vi "Run Till Abort TESTES.vi"() -> ()   [LabVIEW 2012]
uses:
  CCDCamera/CCDCamera.lvclass
  <userlib>/atmcd32d.llb/TriggerMode_mode typedef.ctl
  <userlib>/atmcd32d.llb/HSSpeed_type typedef.ctl
  <userlib>/atmcd32d.llb/Shutter_type typedef.ctl
  <userlib>/atmcd32d.llb/Shutter_mode typedef.ctl
  <userlib>/atmcd32d.llb/ReadMode_mode typedef.ctl
  <userlib>/atmcd32d.llb/AcquisitionMode_mode typedef.ctl
panel:
  out "exposure":sgl format="%.2f"
  out "kinetic":sgl format="%.2f"
  in  "stop":bool
  out "size(s) 2":i32
  out "index":i32
  out "array":u16[](array[numeric])
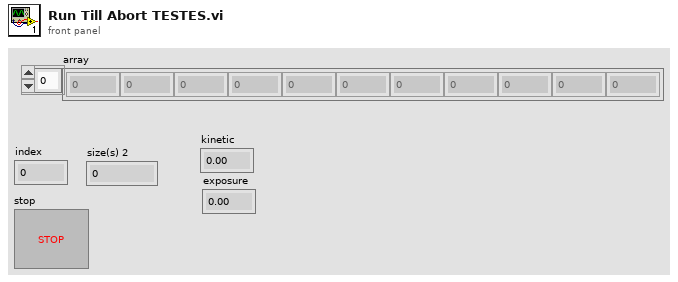
[diagram p1: front panel]
types:
  T1 = typedef "ReadMode_mode typedef.ctl" = enum16{"Full Vertical Binning", "Multi-Track", "Random-Track", "Single-Track", "Image"}
  T2 = typedef "Shutter_mode typedef.ctl" = enum16{"Auto", "Open", "Close", "N/A (3)", "Open FVB Series", "Open Any Series"}
  T3 = typedef "Shutter_type typedef.ctl" = enum16{"TTL Low", "TTL High"}
  T4 = typedef "HSSpeed_type typedef.ctl" = enum16{"EM Amp", "Conventional Amp"}
  T5 = typedef "TriggerMode_mode typedef.ctl" = enum16{"Internal", "External", "N/A (2)", "N/A (3)", "N/A (4)", "N/A (5)", "External Start", "External Exposure (Bulb)", "N/A (8)", "External FVB EM", "Software", "N/A (11)", "External Charge Shifting"}
  T6 = typedef "AcquisitionMode_mode typedef.ctl" = enum16{"Reserved (0)", "Single Scan", "Accumulate", "Kinetics", "Fast Kinetics", "Run Till Abort", "Reserved (6)", "Reserved (7)", "Reserved (8)", "Time Delayed Integration"}
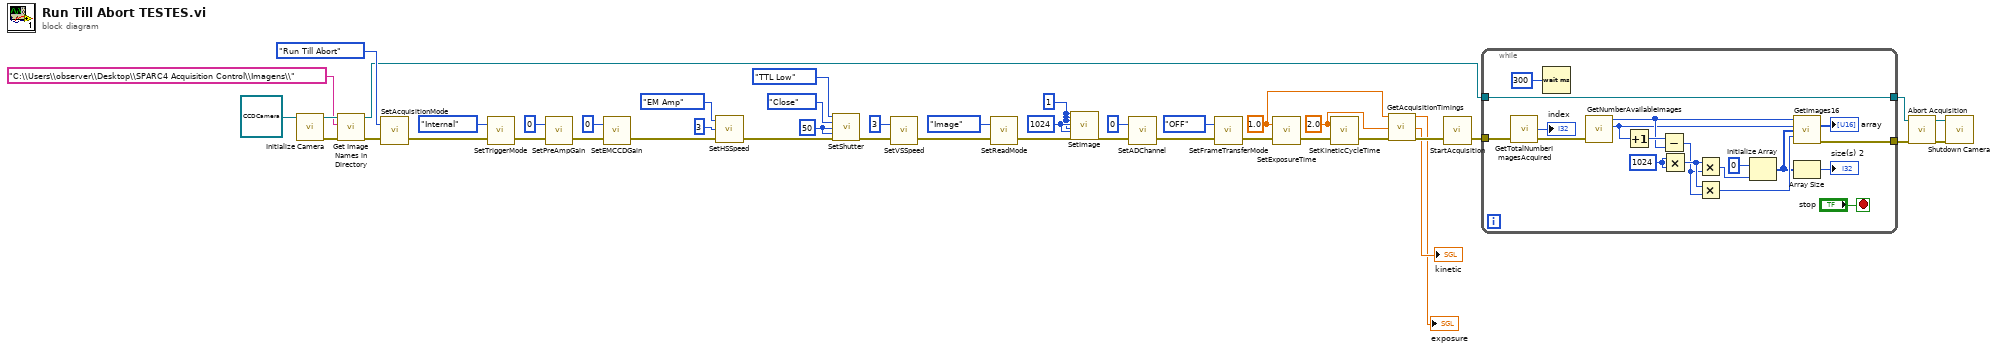
[diagram p0: block diagram]
diagram:
  w3 = sgl 2.0 ("kinetic input")
  w4 = sgl 1.0 ("exposure input")
  w21 = 1024 ("hbin")
  w14 = 1 ("hbin")
  w24 = 50 ("closingtime")
  n1 = call "Initialize Camera.vi"("CCDCamera in"=refnum<class "CCDCamera.lvclass"> refnum) -> ("error out"=w18:errorcluster, "CCDCamera out"=w17:refnum<class "CCDCamera.lvclass">)  [unwired: 9 in]
  n2 = call "Get Image Names in Directory.vi"("error in (no error)"=w18, "Image Path"="C:\\Users\\observer\\Desktop\\SPARC4 Acquisition Control\\Imagens\\", "CCDCamera in"=w17) -> ("error out"=w15:errorcluster, "CCDCamera out"=w12:refnum<class "CCDCamera.lvclass">)  [unwired: 7 in]
  n3 = call <userlib>:"SetAcquisitionMode.vi"("error in (no error)"=w15, "mode"=AcquisitionMode_mode_typedef."Run Till Abort") -> ("error out"=w42:errorcluster)  [unwired: 1 out]
  n4 = call <userlib>:"SetTriggerMode.vi"("error in (no error)"=w42, "mode"=TriggerMode_mode_typedef."Internal") -> ("error out"=w36:errorcluster)  [unwired: 1 out]
  n5 = call <userlib>:"SetPreAmpGain.vi"("error in (no error)"=w36, "index"=0) -> ("error out"=w34:errorcluster)  [unwired: 1 out]
  n6 = call <userlib>:"SetEMCCDGain.vi"("error in (no error)"=w34, "gain"=0) -> ("error out"=w35:errorcluster)  [unwired: 1 out]
  n7 = call <userlib>:"SetHSSpeed.vi"("error in (no error)"=w35, "index"=3, "type"=HSSpeed_type_typedef."EM Amp") -> ("error out"=w37:errorcluster)  [unwired: 1 in, 1 out]
  n8 = call <userlib>:"SetShutter.vi"("type"=Shutter_type_typedef."TTL Low", "mode"=Shutter_mode_typedef."Close", "closingtime"=w24, "openingtime"=w24, "error in (no error)"=w37) -> ("error out"=w41:errorcluster)  [unwired: 9 in, 1 out]
  n9 = call <userlib>:"SetVSSpeed.vi"("error in (no error)"=w41, "index"=3) -> ("error out"=w40:errorcluster)  [unwired: 1 out]
  n10 = call <userlib>:"SetReadMode.vi"("error in (no error)"=w40, "mode"=ReadMode_mode_typedef."Image") -> ("error out"=w39:errorcluster)  [unwired: 1 out]
  n11 = call <userlib>:"SetImage.vi"("hbin"=w14, "vbin"=w14, "hstart"=w14, "hend"=w21, "vstart"=w14, "vend"=w21, "error in (no error)"=w39) -> ("error out"=w38:errorcluster)  [unwired: 19 in, 1 out]
  n12 = call <userlib>:"SetADChannel.vi"("error in (no error)"=w38, "channel"=0) -> ("error out"=w33:errorcluster)  [unwired: 1 out]
  n13 = call <userlib>:"SetFrameTransferMode.vi"("error in (no error)"=w33, "mode"=enum16{"OFF", "ON"}."OFF") -> ("error out"=w13:errorcluster)  [unwired: 1 out]
  n14 = call <userlib>:"SetExposureTime.vi"("error in (no error)"=w13, "time"=w4) -> ("error out"=w19:errorcluster)  [unwired: 1 out]
  n15 = call <userlib>:"SetKineticCycleTime.vi"("error in (no error)"=w19, "time"=w3) -> ("error out"=w6:errorcluster)  [unwired: 1 out]
  n16 = call <userlib>:"GetAcquisitionTimings.vi"("exposure input"=w4, "kinetic input"=w3, "error in (no error)"=w6) -> ("exposure"=→"exposure":sgl, "kinetic"=→"kinetic":sgl, "error out"=w5:errorcluster)  [unwired: 8 in, 2 out]
  n17 = call <userlib>:"StartAcquisition.vi"("error in (no error)"=w5) -> ("error out"=w9:errorcluster)  [unwired: 1 in, 1 out]
  n18 = while {
    tunnel: w9 -> [w62]
    tunnel: [w60] -> w8
    tunnel: w12 -> [w60]
    tunnel: [w54] -> w7
    stop <- "stop" stop-if-true
    w56 = 1024
    n19 = call <userlib>:"GetTotalNumberImagesAcquired.vi"("error in (no error)"=w62) -> ("error out"=w55:errorcluster, "index"=→"index":i32)  [unwired: 2 in, 1 out]
    n20 = Wait (ms)(milliseconds to wait=u32 300) -> ()  [unwired: 1 out]
    n21 = call <userlib>:"GetNumberAvailableImages.vi"("error in (no error)"=w55) -> ("first"=w47:i32, "last"=w46:i32)  [unwired: 2 in, 2 out]
    n22 = Increment(x=w46) -> (x+1=w57:i32)
    n23 = Subtract(x=w57, y=w47) -> (x-y=w45:i32)
    n24 = Multiply(x=w56, y=w56) -> (x*y=w53:i32)
    n25 = Multiply(x=w53, y=w45) -> (x*y=w51:i32)
    n26 = Multiply(x=w53, y=w45) -> (x*y=w58:i32)
    n27 = Initialize Array(u16 0, w51) -> (w50:u16[])
    n28 = call <userlib>:"GetImages16.vi"("first"=w47, "last"=w46, "array"=w50, "size"=w58) -> ("array"=→"array":u16[], "error out"=w54:errorcluster)  [unwired: 7 in, 3 out]
    n29 = Array Size(array=w50) -> (size(s)=→"size(s) 2":i32)
  }
  n30 = call "Abort Acquisition.vi"("error in (no error)"=w7, "CCDCamera in"=w8) -> ("error out"=w10:errorcluster, "CCDCamera out"=w11:refnum<class "CCDCamera.lvclass">)  [unwired: 8 in]
  n31 = call "Shutdown Camera.vi"("error in (no error)"=w10, "CCDCamera in"=w11) -> ()  [unwired: 8 in, 2 out]
